vi "kvCanSetBusParamsFd.vi"(0 "Channel Handle (input only)":i32, 1 "Frequency":i32, 2 "Time Segment 1":u32, 3 "Time Segment 2":u32, 4 "Synchronization Jump Width":u32, 5 "error in (no error)":errorcluster) -> (14 "Channel Handle (output only)":i32, 19 "error out":errorcluster)   [LabVIEW 2023]
doc: "This function sets the data phase bus timing parameters for the specified CAN controller.\n\nThe library provides default values for Time Segment 1, Time Segment 2 and Synchronization Jump Width when Frequency is specified to one of the pre-defined FD constants in the kvCanTranslateBaud.ctl.\n\nIf frequency is any other value, no default values are supplied by the library."
uses:
  canlib32.dll
panel:
  # "Bus Parameters to be used by a CAN FD  channel for the transmission\nof the data bytes when the message flag indicate bit rate switch."
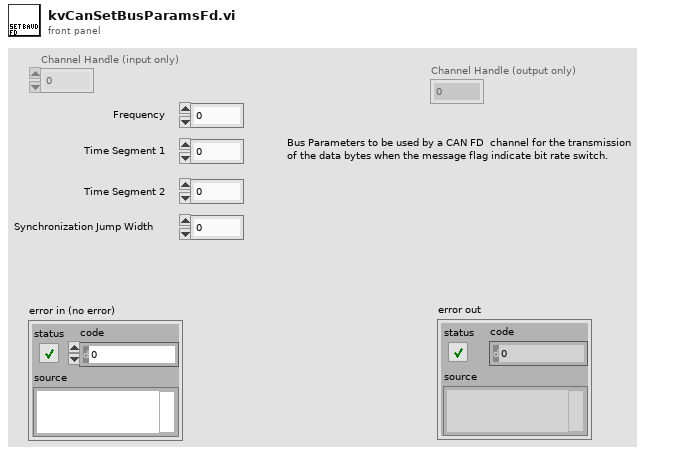
[diagram p1: front panel]
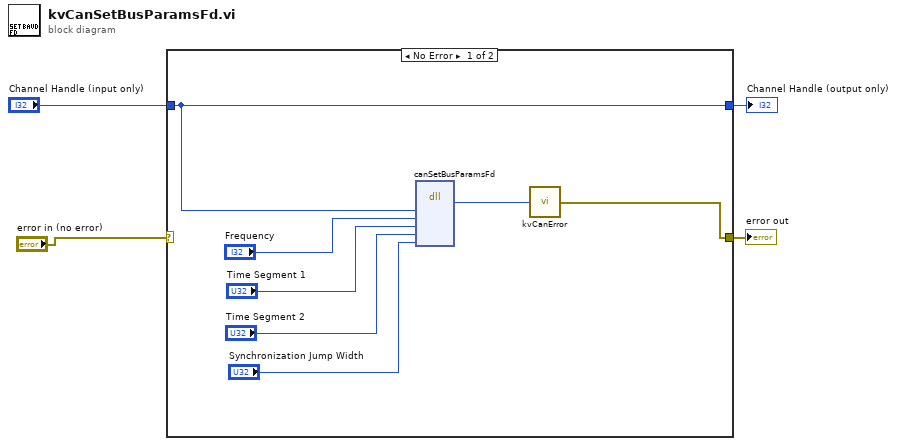
[diagram p0: block diagram]
diagram:
  n1 = case shown="No Error" "error in (no error)" {
    selector: "error in (no error)" -> [_ w13]
    tunnel: [w9 w13] -> w3
    tunnel: "Channel Handle (input only)" -> [w11 w12]
    tunnel: [w11 w12] -> w1
    frame No Error {
      n2 = dll-call lib="canlib32.dll" fn="canSetBusParamsFd"("handle"=w11, "freq"="Frequency", "tseg1"="Time Segment 1", "tseg2"="Time Segment 2", "sjw"="Synchronization Jump Width") -> ("return type"=w10:i32)  [unwired: 8 in, 2 out]
      n3 = call "kvCanError.vi"("error code"=w10) -> ("error out"=w9:errorcluster)
    }
    frame Error {
    }
  }
  "error out" <- w3
  "Channel Handle (output only)" <- w1
